vi "lvstyx_read_all_path_bin.vi"(8 "error in (no error)":errorcluster, 9 "path":string, 10 "lim":i32=2048, 11 "client ptr":u32) -> (0 "error out":errorcluster, 2 "buf":u8[](array[numeric]), 3 "dup client ptr":u32)   [LabVIEW 2010, in "lib1299.lvlib"]
uses:
  lib1299.lvlib
  cstyx/win32/cstyx.dll
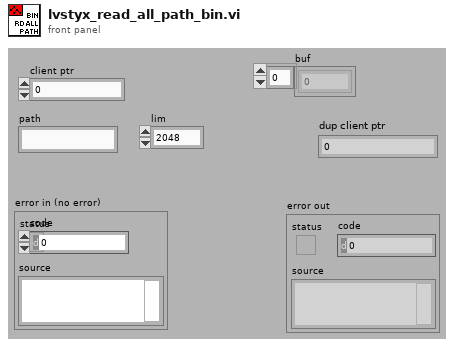
[diagram p1: front panel]
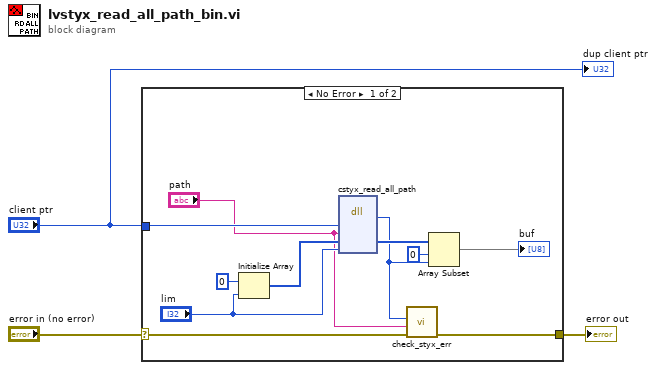
[diagram p0: block diagram]
diagram:
  n1 = case shown="No Error" "error in (no error)" {
    selector: "error in (no error)" -> [w11 w15]
    tunnel: "client ptr" -> [w12 _]
    tunnel: [w10 w15] -> w3
    frame No Error {
      n2 = Initialize Array(i8 0 ("element"), "lim") -> (w9:i8[])
      n3 = dll-call lib="C:/work/ads1299evm/lib_1299/Styx/cstyx/win32/cstyx.dll" fn="cstyx_read_all_path"("client"=w12, "path"="path", "buf"=w9, "lim"="lim") -> (w6:i32, "buf"=w8:i8[])  [unwired: 6 in, 2 out]
      n4 = call "check_styx_err.vi"("error in (no error)"=w11, "Additional Comment"="path", "return val"=w6) -> ("error out"=w10:errorcluster)  [unwired: 8 in]
      n5 = Array Subset(array=w8, index=0, length=w6) -> (→"buf":i8[])
    }
    frame Error {
    }
  }
  "error out" <- w3
  "dup client ptr" <- "client ptr"
